vi "angle_deviation_corrector.vi"(0 "angle":dbl, 2 "angle 2":dbl, 3 "angle 3":dbl) -> (6 "angle corrected":dbl, 7 "angle corrected 2":dbl, 9 "angle corrected 3":dbl)   [LabVIEW 2019]
panel:
  # "Angle deviation corrector"
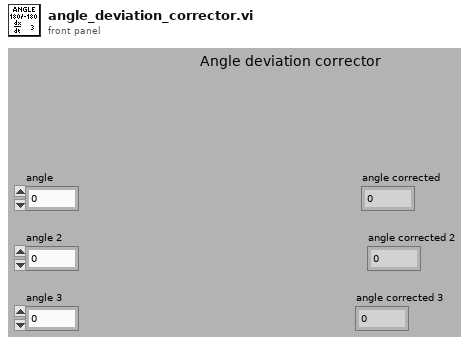
[diagram p1: front panel]
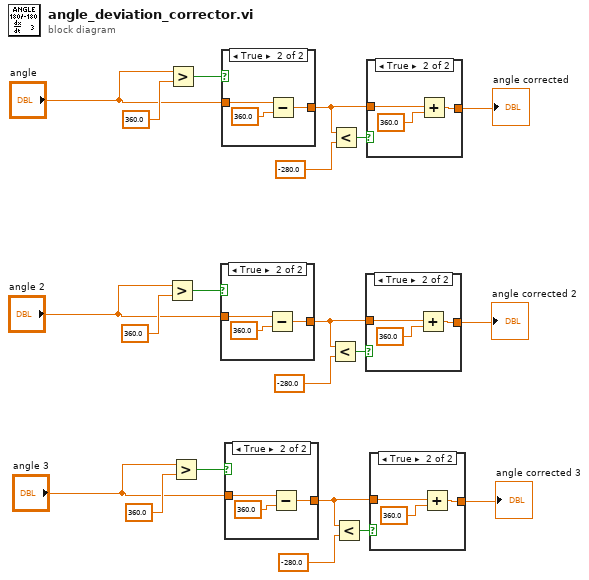
[diagram p0: block diagram]
diagram:
  n1 = Greater?(x="angle 2", y=360.0) -> (0:w12:bool)
  n2 = Greater?(x="angle", y=360.0) -> (0:w19:bool)
  n3 = Greater?(x="angle 3", y=360.0) -> (0:w5:bool)
  n4 = case shown="True" w12 {
    tunnel: "angle 2" -> [w22 w24]
    tunnel: [w22 w23] -> w10
    frame False {
    }
    frame True {
      n5 = Subtract(x=w24, y=360.0) -> (x-y=w23:dbl)
    }
  }
  n6 = case shown="True" w19 {
    tunnel: "angle" -> [w26 w28]
    tunnel: [w26 w27] -> w17
    frame False {
    }
    frame True {
      n7 = Subtract(x=w28, y=360.0) -> (x-y=w27:dbl)
    }
  }
  n8 = case shown="True" w5 {
    tunnel: "angle 3" -> [w30 w32]
    tunnel: [w30 w31] -> w3
    frame False {
    }
    frame True {
      n9 = Subtract(x=w32, y=360.0) -> (x-y=w31:dbl)
    }
  }
  n10 = Less?(x=w10, y=-280.0) -> (x < y?=w11:bool)
  n11 = Less?(x=w17, y=-280.0) -> (x < y?=w18:bool)
  n12 = Less?(x=w3, y=-280.0) -> (x < y?=w4:bool)
  n13 = case shown="True" w11 {
    tunnel: w10 -> [w34 w36]
    tunnel: [w34 w35] -> w8
    frame False {
    }
    frame True {
      n14 = Add(x=w36, y=360.0) -> (x+y=w35:dbl)
    }
  }
  "angle corrected 2" <- w8
  n15 = case shown="True" w18 {
    tunnel: w17 -> [w38 w40]
    tunnel: [w38 w39] -> w15
    frame False {
    }
    frame True {
      n16 = Add(x=w40, y=360.0) -> (x+y=w39:dbl)
    }
  }
  "angle corrected" <- w15
  n17 = case shown="True" w4 {
    tunnel: w3 -> [w42 w44]
    tunnel: [w42 w43] -> w1
    frame False {
    }
    frame True {
      n18 = Add(x=w44, y=360.0) -> (x+y=w43:dbl)
    }
  }
  "angle corrected 3" <- w1
